vi "Load Config_Folder Name Edit.vi"(8 "error in (no error)":errorcluster, 11 "Refnum in":T2) -> (0 "error out":errorcluster, 2 "Folder Name Edit":T1, 3 "Refnum out":T2)   [LabVIEW 2019, in "AutoMenuCreator.lvlib"]
uses:
  AutoMenuCreator.lvlib
  <vilib>/Utility/config.llb/Config Data RefNum.ctl
  Ctl/Ctl_Config_Folder Name Edit.ctl
  <vilib>/Utility/config.llb/NI_LVConfig.lvlib
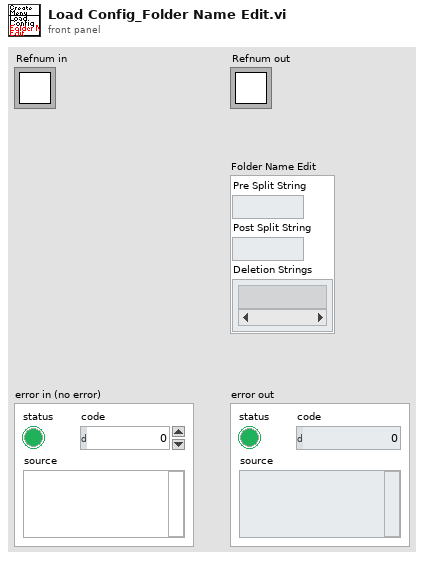
[diagram p1: front panel]
types:
  T1 = typedef "AutoMenuCreator.lvlib/Ctl_Config_Folder Name Edit.ctl" = cluster{"Pre Split String":string, "Post Split String":string, "Deletion Strings":string[]}
  T2 = typedef "NI_LVConfig.lvlib/Config Data RefNum.ctl" = refnum<k1>
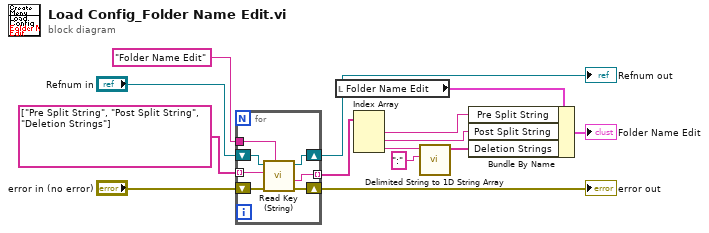
[diagram p0: block diagram]
diagram:
  n1 = for {
    tunnel: "Folder Name Edit" ("section") -> [w19]
    shift-right: [w18] -> w10
    shift-left: "Refnum in" -> [w20]
    shift-right: [w17] -> w9
    shift-left: "error in (no error)" -> [w21]
    tunnel: string[] ["Pre Split String", "Post Split String", "Deletion Strings"] ("key") -> [w16] mode=indexing
    tunnel: [w15] -> w8 mode=indexing
    n2 = call <vilib>:"Read Key (String).vi"("section"=w19, "error in (no error)"=w21, "key"=w16, "refnum"=w20) -> ("error out"=w17:errorcluster, "value"=w15:string, "refnum out"=w18:T2)  [unwired: 4 in, 1 out]
  }
  "error out" <- w9
  "Refnum out" <- w10
  n3 = local read "Folder Name Edit"() -> (w4:T1)
  n4 = Index Array(array=w8) -> (element #1=w6:string, element #2=w7:string, element #3=w2:string)  [unwired: 3 in]
  n5 = call <vilib>:"Delimited String to 1D String Array.vi"("delimiter"=":", "delimited string"=w2) -> ("string array"=w1:string[])  [unwired: 9 in]
  n6 = Bundle By Name(cluster=w4, "Pre Split String"=w6, "Post Split String"=w7, "Deletion Strings"=w1) -> (→"Folder Name Edit":T1)
